vi "csuClose.vi"   [LabVIEW 2017]
uses:
  globalDevices.vi
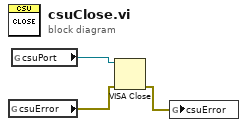
[diagram p0: block diagram]
diagram:
  n1 = global read "globalDevices.vi" "csuError"() -> (w2:errorcluster)
  n2 = global read "globalDevices.vi" "csuPort"() -> (w3:refnum<visa-resource-name>)
  n3 = VISA Close(VISA resource name=w3, error in (no error)=w2) -> (error out=w1:errorcluster)
  n4 = global write "globalDevices.vi" "csuError"(w1) -> ()
